vi "Run.vi"(8 "error in (no error)":errorcluster, 11 "Channel in":refnum<class "Channel.lvclass">) -> (0 "error out":errorcluster, 3 "Channel out":refnum<class "Channel.lvclass">)   [LabVIEW 2018, in "Channel.lvclass"]
uses:
  Channel.lvclass
  Channel.lvclass/Channel.ctl
  CCDCamera/CCDCamera.lvclass/CCDCamera.ctl
  State Machine/State Machine.lvclass
  Image Constructor/Image Constructor.lvclass
  CCDCamera/CCDCamera.lvclass
  Save Image/Save Image.lvclass
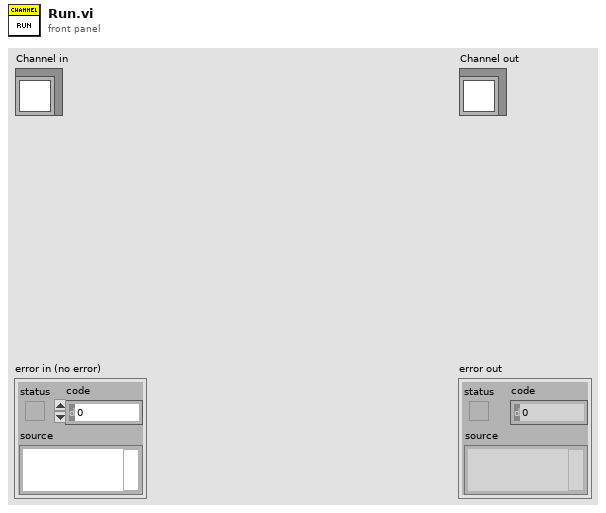
[diagram p1: front panel]
types:
  T1 = cluster{"Acquiring":bool, "% Acquired":u16, "STATUS":string}
  T2 = cluster{"Exposure Time":sgl, "Pre-amp gain":u8, "Readout Rate":u8, "EM Mode":u8, "EM Gain":u16, "Binning":u16, "Initial Line":u16, "Initial Cloumn":u16, "Final Line":u16, "Final Column":u16, "Kinetic Series Length":u32, "Shutter Mode":u8, "Cooler ON/OFF":u8, "Temperature":i8, "Image Name":string, "Image Path":string, "Current Temperature":i16, "Temperatue Status":string, "Serial Number":u16, " #image":u32}
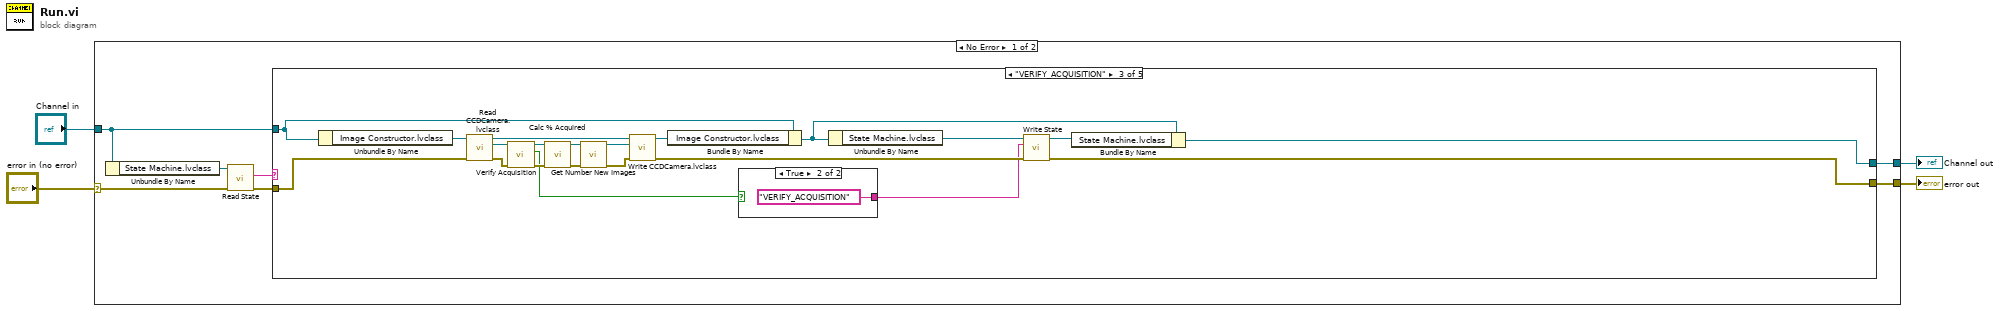
[diagram p0: block diagram]
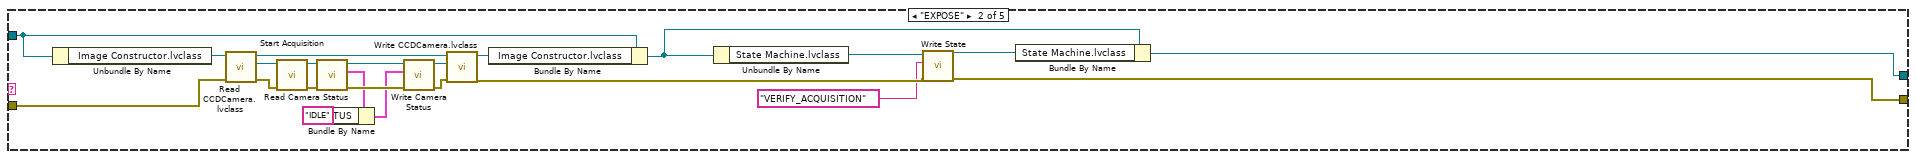
[diagram p3: hidden frame]
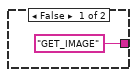
[diagram p4: hidden frame]
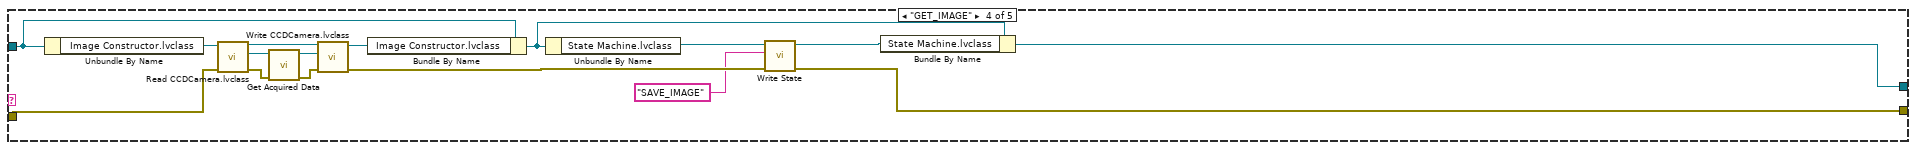
[diagram p5: hidden frame]
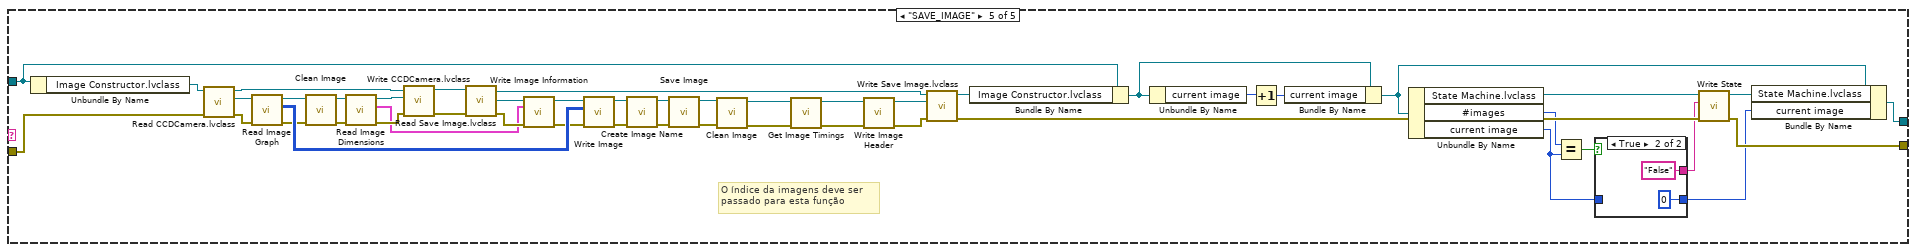
[diagram p6: hidden frame]
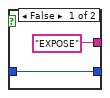
[diagram p7: hidden frame]
diagram:
  n1 = case shown="No Error" "error in (no error)" {
    selector: "error in (no error)" -> [w7 w129]
    tunnel: [w11 w129] -> w3
    tunnel: [w9 w128] -> w1
    tunnel: "Channel in" -> [w10 w128]
    frame No Error {
      n2 = Unbundle By Name(w10) -> ("State Machine.lvclass"=w8:refnum<class "State Machine.lvclass">)
      n3 = call-dynamic "Read State.vi"("error in (no error)"=w7, "State Machine in"=w8) -> ("error out"=w6:errorcluster, "State"=w5:string)  [unwired: 7 in, 1 out]
      n4 = case shown="\"VERIFY_ACQUISITION\"" w5 {
        tunnel: w6 -> [w13 w33 w55 w71 w123]
        tunnel: [w13 w25 w43 w61 w89] -> w11
        tunnel: [w12 w28 w47 w68 w86] -> w9
        tunnel: w10 -> [w12 w31 w52 w66 w112]
        frame "False", Default {
        }
        frame "EXPOSE" {
          n5 = Unbundle By Name(w31) -> ("Image Constructor.lvclass"=w32:refnum<class "Image Constructor.lvclass">)
          n6 = call "Read CCDCamera.lvclass.vi"("error in (no error)"=w33, "Image Constructor in"=w32) -> ("error out"=w35:errorcluster, "CCDCamera.lvclass"=w34:refnum<class "CCDCamera.lvclass">, "Image Constructor out"=w36:refnum<class "Image Constructor.lvclass">)  [unwired: 7 in]
          n7 = call "Start Acquisition.vi"("error in (no error)"=w35, "CCDCamera in"=w34) -> ("error out"=w21:errorcluster, "CCDCamera out"=w22:refnum<class "CCDCamera.lvclass">)  [unwired: 8 in]
          n8 = call "Read Camera Status.vi"("error in (no error)"=w21, "CCDCamera in"=w22) -> ("error out"=w19:errorcluster, "Camera Status"=w15:T1, "CCDCamera out"=w20:refnum<class "CCDCamera.lvclass">)  [unwired: 7 in]
          n9 = Bundle By Name(cluster=w15, "STATUS"="IDLE") -> (w16:T1)
          n10 = call "Write Camera Status.vi"("error in (no error)"=w19, "Camera Status"=w16, "CCDCamera in"=w20) -> ("error out"=w17:errorcluster, "CCDCamera out"=w18:refnum<class "CCDCamera.lvclass">)  [unwired: 7 in]
          n11 = call "Write CCDCamera.lvclass.vi"("error in (no error)"=w17, "CCDCamera.lvclass"=w18, "Image Constructor in"=w36) -> ("error out"=w24:errorcluster, "Image Constructor out"=w30:refnum<class "Image Constructor.lvclass">)  [unwired: 7 in]
          n12 = Bundle By Name(cluster=w31, "Image Constructor.lvclass"=w30) -> (w29:refnum<class "Channel.lvclass">)
          n13 = Unbundle By Name(w29) -> ("State Machine.lvclass"=w26:refnum<class "State Machine.lvclass">)
          n14 = call-dynamic "Write State.vi"("error in (no error)"=w24, "State"="VERIFY_ACQUISITION", "State Machine in"=w26) -> ("error out"=w25:errorcluster, "State Machine out"=w27:refnum<class "State Machine.lvclass">)  [unwired: 7 in]
          n15 = Bundle By Name(cluster=w29, "State Machine.lvclass"=w27) -> (w28:refnum<class "Channel.lvclass">)
        }
        frame "VERIFY_ACQUISITION" {
          n16 = Unbundle By Name(w52) -> ("Image Constructor.lvclass"=w53:refnum<class "Image Constructor.lvclass">)
          n17 = call "Read CCDCamera.lvclass.vi"("error in (no error)"=w55, "Image Constructor in"=w53) -> ("error out"=w57:errorcluster, "CCDCamera.lvclass"=w56:refnum<class "CCDCamera.lvclass">, "Image Constructor out"=w54:refnum<class "Image Constructor.lvclass">)  [unwired: 7 in]
          n18 = call "Verify Acquisition.vi"("error in (no error)"=w57, "CCDCamera in"=w56) -> ("error out"=w49:errorcluster, "Acquiring"=w37:bool, "CCDCamera out"=w48:refnum<class "CCDCamera.lvclass">)  [unwired: 7 in]
          n19 = call "Calc % Acquired.vi"("error in (no error)"=w49, "CCDCamera in"=w48) -> ("error out"=w40:errorcluster, "CCDCamera out"=w41:refnum<class "CCDCamera.lvclass">)  [unwired: 8 in]
          n20 = call "Get Number New Images.vi"("error in (no error)"=w40, "CCDCamera in"=w41) -> ("error out"=w38:errorcluster, "CCDCamera out"=w39:refnum<class "CCDCamera.lvclass">)  [unwired: 7 in, 1 out]
          n21 = call "Write CCDCamera.lvclass.vi"("error in (no error)"=w38, "CCDCamera.lvclass"=w39, "Image Constructor in"=w54) -> ("error out"=w44:errorcluster, "Image Constructor out"=w51:refnum<class "Image Constructor.lvclass">)  [unwired: 7 in]
          n22 = Bundle By Name(cluster=w52, "Image Constructor.lvclass"=w51) -> (w50:refnum<class "Channel.lvclass">)
          n23 = case shown="True" w37 {
            tunnel: ["GET_IMAGE" "VERIFY_ACQUISITION"] -> w42
            frame False {
            }
            frame True {
            }
          }
          n24 = Unbundle By Name(w50) -> ("State Machine.lvclass"=w46:refnum<class "State Machine.lvclass">)
          n25 = call-dynamic "Write State.vi"("error in (no error)"=w44, "State"=w42, "State Machine in"=w46) -> ("error out"=w43:errorcluster, "State Machine out"=w45:refnum<class "State Machine.lvclass">)  [unwired: 7 in]
          n26 = Bundle By Name(cluster=w50, "State Machine.lvclass"=w45) -> (w47:refnum<class "Channel.lvclass">)
        }
        frame "GET_IMAGE" {
          n27 = Unbundle By Name(w66) -> ("Image Constructor.lvclass"=w70:refnum<class "Image Constructor.lvclass">)
          n28 = call "Read CCDCamera.lvclass.vi"("error in (no error)"=w71, "Image Constructor in"=w70) -> ("error out"=w73:errorcluster, "CCDCamera.lvclass"=w72:refnum<class "CCDCamera.lvclass">, "Image Constructor out"=w75:refnum<class "Image Constructor.lvclass">)  [unwired: 7 in]
          n29 = call "Get Acquired Data.vi"("error in (no error)"=w73, "CCDCamera in"=w72) -> ("error out"=w74:errorcluster, "CCDCamera out"=w67:refnum<class "CCDCamera.lvclass">)  [unwired: 8 in]
          n30 = call "Write CCDCamera.lvclass.vi"("error in (no error)"=w74, "CCDCamera.lvclass"=w67, "Image Constructor in"=w75) -> ("error out"=w62:errorcluster, "Image Constructor out"=w69:refnum<class "Image Constructor.lvclass">)  [unwired: 7 in]
          n31 = Bundle By Name(cluster=w66, "Image Constructor.lvclass"=w69) -> (w65:refnum<class "Channel.lvclass">)
          n32 = Unbundle By Name(w65) -> ("State Machine.lvclass"=w63:refnum<class "State Machine.lvclass">)
          n33 = call-dynamic "Write State.vi"("error in (no error)"=w62, "State"="SAVE_IMAGE", "State Machine in"=w63) -> ("error out"=w61:errorcluster, "State Machine out"=w64:refnum<class "State Machine.lvclass">)  [unwired: 7 in]
          n34 = Bundle By Name(cluster=w65, "State Machine.lvclass"=w64) -> (w68:refnum<class "Channel.lvclass">)
        }
        frame "SAVE_IMAGE" {
          # "O índice da imagens deve ser \npassado para esta função"
          n35 = Unbundle By Name(w112) -> ("Image Constructor.lvclass"=w88:refnum<class "Image Constructor.lvclass">)
          n36 = call "Read CCDCamera.lvclass.vi"("error in (no error)"=w123, "Image Constructor in"=w88) -> ("error out"=w121:errorcluster, "CCDCamera.lvclass"=w122:refnum<class "CCDCamera.lvclass">, "Image Constructor out"=w114:refnum<class "Image Constructor.lvclass">)  [unwired: 7 in]
          n37 = call "Read Image Graph.vi"("error in (no error)"=w121, "CCDCamera in"=w122) -> ("error out"=w117:errorcluster, "Image Graph"=w120:u16[][][], "CCDCamera out"=w118:refnum<class "CCDCamera.lvclass">)  [unwired: 7 in]
          n38 = call "Clean Image.vi"("error in (no error)"=w117, "CCDCamera in"=w118) -> ("error out"=w107:errorcluster, "CCDCamera out"=w106:refnum<class "CCDCamera.lvclass">)  [unwired: 8 in]
          n39 = call "Read Image Dimensions.vi"("error in (no error)"=w107, "CCDCamera in"=w106) -> ("error out"=w104:errorcluster, "CCD Config"=w87:T2, "CCDCamera out"=w105:refnum<class "CCDCamera.lvclass">)  [unwired: 7 in]
          n40 = call "Write CCDCamera.lvclass.vi"("error in (no error)"=w104, "CCDCamera.lvclass"=w105, "Image Constructor in"=w114) -> ("error out"=w116:errorcluster, "Image Constructor out"=w115:refnum<class "Image Constructor.lvclass">)  [unwired: 7 in]
          n41 = call "Read Save Image.lvclass.vi"("error in (no error)"=w116, "Image Constructor in"=w115) -> ("error out"=w100:errorcluster, "Save Image.lvclass"=w101:refnum<class "Save Image.lvclass">, "Image Constructor out"=w119:refnum<class "Image Constructor.lvclass">)  [unwired: 7 in]
          n42 = call "Write Image Information.vi"("error in (no error)"=w100, "CCD Config"=w87, "Save Image in"=w101) -> ("error out"=w103:errorcluster, "Save Image out"=w102:refnum<class "Save Image.lvclass">)  [unwired: 7 in]
          n43 = call "Write Image.vi"("error in (no error)"=w103, "Image"=w120, "Save Image in"=w102) -> ("error out"=w109:errorcluster, "Save Image out"=w110:refnum<class "Save Image.lvclass">)  [unwired: 7 in]
          n44 = call "Create Image Name.vi"("error in (no error)"=w109, "Save Image in"=w110) -> ("error out"=w108:errorcluster, "Save Image out"=w111:refnum<class "Save Image.lvclass">)  [unwired: 8 in]
          n45 = call "Save Image.vi"("error in (no error)"=w108, "Save Image in"=w111) -> ("error out"=w98:errorcluster, "Save Image out"=w99:refnum<class "Save Image.lvclass">)  [unwired: 8 in]
          n46 = call "Clean Image.vi"("error in (no error)"=w98, "Save Image in"=w99) -> ("error out"=w96:errorcluster, "Save Image out"=w97:refnum<class "Save Image.lvclass">)  [unwired: 8 in]
          n47 = call "Get Image Timings.vi"("error in (no error)"=w96, "Save Image in"=w97) -> ("error out"=w95:errorcluster, "Save Image out"=w94:refnum<class "Save Image.lvclass">)  [unwired: 8 in]
          n48 = call "Write Image Header.vi"("error in (no error)"=w95, "Save Image in"=w94) -> ("error out"=w92:errorcluster, "Save Image out"=w93:refnum<class "Save Image.lvclass">)  [unwired: 8 in]
          n49 = call "Write Save Image.lvclass.vi"("error in (no error)"=w92, "Save Image.lvclass"=w93, "Image Constructor in"=w119) -> ("error out"=w85:errorcluster, "Image Constructor out"=w113:refnum<class "Image Constructor.lvclass">)  [unwired: 7 in]
          n50 = Bundle By Name(cluster=w112, "Image Constructor.lvclass"=w113) -> (w84:refnum<class "Channel.lvclass">)
          n51 = Unbundle By Name(w84) -> ("current image"=w82:u32)
          n52 = Increment(x=w82) -> (x+1=w81:u32)
          n53 = Bundle By Name(cluster=w84, "current image"=w81) -> (w83:refnum<class "Channel.lvclass">)
          n54 = Unbundle By Name(w83) -> ("State Machine.lvclass"=w90:refnum<class "State Machine.lvclass">, "#images"=w80:u32, "current image"=w76:u32)
          n55 = Equal?(x=w80, y=w76) -> (x = y?=w79:bool)
          n56 = case shown="True" w79 {
            tunnel: ["EXPOSE" "False"] -> w78
            tunnel: [w124 u32 0 ("current image")] -> w77
            tunnel: w76 -> [w124 _]
            frame False {
            }
            frame True {
            }
          }
          n57 = call-dynamic "Write State.vi"("error in (no error)"=w85, "State"=w78, "State Machine in"=w90) -> ("error out"=w89:errorcluster, "State Machine out"=w91:refnum<class "State Machine.lvclass">)  [unwired: 7 in]
          n58 = Bundle By Name(cluster=w83, "State Machine.lvclass"=w91, "current image"=w77) -> (w86:refnum<class "Channel.lvclass">)
        }
      }
    }
    frame Error {
    }
  }
  "error out" <- w3
  "Channel out" <- w1
